vi "parallel data transfer of sine waves in while loops.vi"() -> ()   [LabVIEW 2020]
uses:
  <extravilib>/ChannelInstances/Stream-dbl/Read With Abort.vi
  <extravilib>/ChannelInstances/Stream-dbl/Write With Abort.vi
  <extravilib>/ChannelInstances/Stream-dbl/EndpointRead.vi
  <extravilib>/ChannelInstances/Stream-dbl/Endpoint.vi
  <extravilib>/ChannelInstances/Stream-dbl/Instantiate.vi
  <extravilib>/ChannelInstances/Stream-dbl/)Channel.vi
  <resource>/ChannelSupport/_ChannelSupport/WaitIfNeeded.vi
  <extravilib>/ChannelInstances/Stream-dbl.lvlib
panel:
  out "Waveform Chart 2":dbl(graph)
  in  "stop":bool
  out "Waveform Chart":dbl(graph)
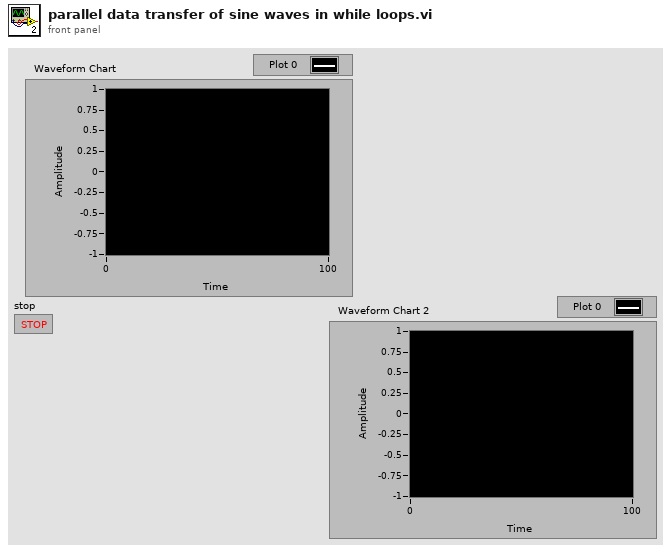
[diagram p1: front panel]
types:
  T1 = typedef "Stream-dbl.lvlib/)Channel.ctl" = refnum<queue>
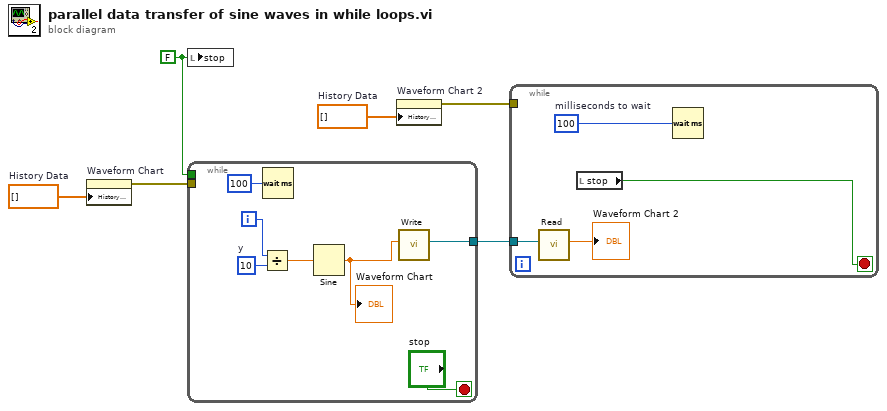
[diagram p0: block diagram]
diagram:
  w4 = FALSE
  w2 = dbl[] []  # History Data
  w6 = dbl[] []  # History Data
  n1 = property on="Waveform Chart" class="WFChart (strict)"("History Data"=w6) -> (error out=w5:errorcluster)  [unwired: 2 in, 1 out]
  n2 = local write "stop"(w4) -> ()
  n3 = while {
    tunnel: w5 -> [_]
    tunnel: w4 -> [_]
    tunnel: [w7] -> w3
    i -> [w13]
    stop <- "stop" stop-if-true
    w12 = 10  # y
    n4 = Divide(x=w13, y=w12) -> (x/y=w11:dbl)
    n5 = Wait (ms)(milliseconds to wait=u32 100) -> ()  [unwired: 1 out]
    n6 = Sine(x=w11) -> (sin(x)=w8:dbl)
    "Waveform Chart" <- w8
    n7 = call <extravilib>:"Write.vi"("element"=w8) -> ("channel"=w7:T1)  [unwired: 8 in, 2 out]
  }
  n8 = property on="Waveform Chart 2" class="WFChart (strict)"("History Data"=w2) -> (error out=w1:errorcluster)  [unwired: 2 in, 1 out]
  n9 = while {
    tunnel: w3 -> [w15]
    tunnel: w1 -> [_]
    stop <- w16 stop-if-true
    w17 = u32 100  # milliseconds to wait
    n10 = call <extravilib>:"Read.vi"("channel"=w15) -> ("element"=→"Waveform Chart 2":dbl)  [unwired: 6 in, 4 out]
    n11 = local read "stop"() -> (w16:bool)
    n12 = Wait (ms)(milliseconds to wait=w17) -> ()  [unwired: 1 out]
  }
